vi "Ch_select.vi"(1 "Device Name":tag="Dev1", 2 "ChB_Source":u16, 3 "ChA_Source":u16) -> (6 "CHBA":tag, 7 "CHAB":tag, 8 "CHB":tag, 9 "CHA":tag)   [LabVIEW 2010]
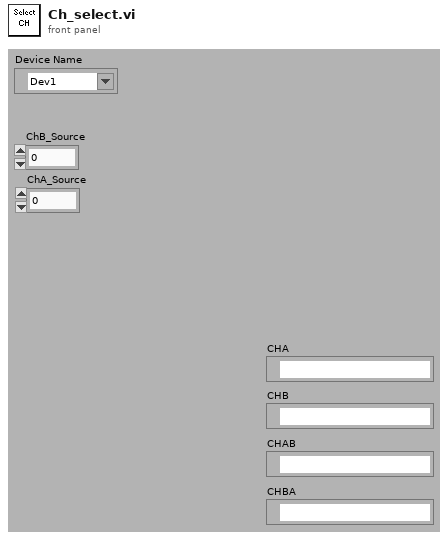
[diagram p1: front panel]
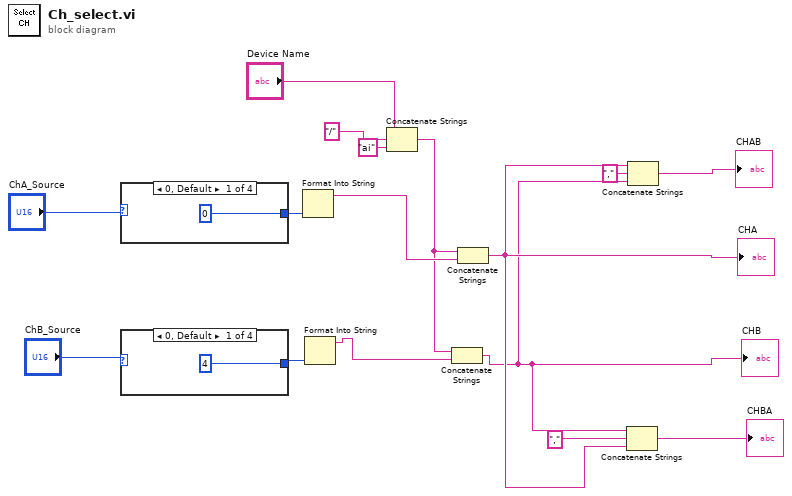
[diagram p0: block diagram]
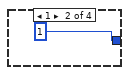
[diagram p2: hidden frame]
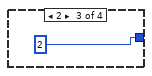
[diagram p3: hidden frame]
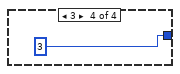
[diagram p4: hidden frame]
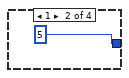
[diagram p5: hidden frame]
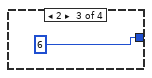
[diagram p6: hidden frame]
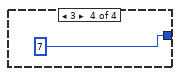
[diagram p7: hidden frame]
diagram:
  n1 = case shown="0, Default" "ChA_Source" {
    tunnel: [0 1 2 3] -> w13
    frame 0, Default {
    }
    frame 1 {
    }
    frame 2 {
    }
    frame 3 {
    }
  }
  n2 = case shown="0, Default" "ChB_Source" {
    tunnel: [4 5 6 7] -> w12
    frame 0, Default {
    }
    frame 1 {
    }
    frame 2 {
    }
    frame 3 {
    }
  }
  n3 = Format Into String(w13) -> (resulting string=w11:string)  [unwired: 3 in, 1 out]
  n4 = Format Into String(w12) -> (resulting string=w9:string)  [unwired: 3 in, 1 out]
  n5 = Concatenate Strings("Device Name", "/" ("string"), "ai" ("string")) -> (w10:string)
  n6 = Concatenate Strings(w10, w9) -> (w5:string)
  "CHB" <- w5
  n7 = Concatenate Strings(w10, w11) -> (w6:string)
  "CHA" <- w6
  n8 = Concatenate Strings(w5, "," ("string"), w6) -> (→"CHBA":string)
  n9 = Concatenate Strings(w6, "," ("string"), w5) -> (→"CHAB":string)
